vi "Write Table Name.vi"(8 "error in (no error)":errorcluster, 10 "Table Name":string, 11 "Import Export in":refnum<class "Export.lvclass">) -> (0 "error out":errorcluster, 3 "Import Export out":refnum<class "Export.lvclass">)   [LabVIEW 2023, in "Data Analysis.lvlib" / "Export.lvlib" / "Export.lvclass"]
uses:
  Export.lvclass
  Export.lvclass/Export.ctl
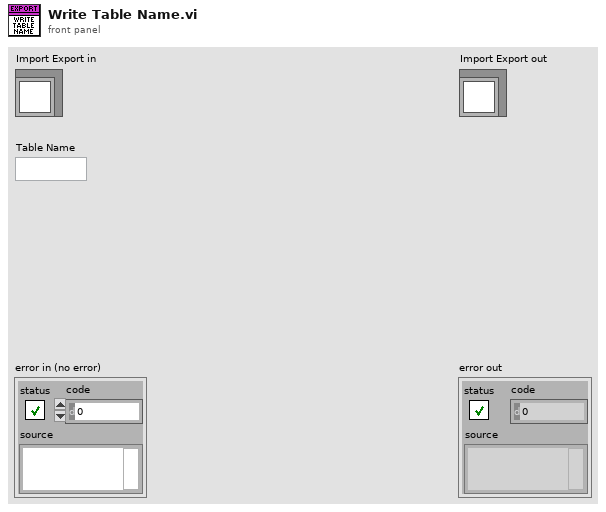
[diagram p1: front panel]
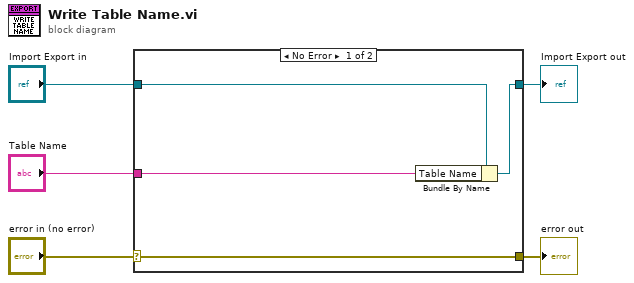
[diagram p0: block diagram]
diagram:
  n1 = case shown="No Error" "error in (no error)" {
    selector: "error in (no error)" -> [w9 w10]
    tunnel: [w9 w10] -> w4
    tunnel: [w7 w11] -> w2
    tunnel: "Import Export in" -> [w8 w11]
    tunnel: "Table Name" -> [w6 _]
    frame No Error {
      n2 = Bundle By Name(cluster=w8, "Table Name"=w6) -> (w7:refnum<class "Export.lvclass">)
    }
    frame Error {
    }
  }
  "error out" <- w4
  "Import Export out" <- w2
